vi "Save Control__A2E.vi"(8 "error in (no error)":errorcluster, 10 "Control VI Type":T1, 11 "vi reference in":refnum<vi>) -> (0 "error out":errorcluster, 3 "vi reference out":refnum<vi>)   [LabVIEW 2021, in "Utilities.lvlib"]
uses:
  ControlTypes__A2E.ctl
  Utilities.lvlib
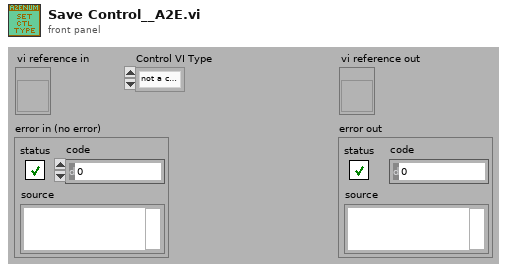
[diagram p1: front panel]
types:
  T1 = typedef "Utilities.lvlib/ControlTypes__A2E.ctl" = enum32{"not a control VI", "control", "typedef", "strict typedef"}
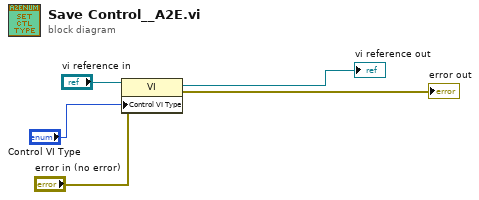
[diagram p0: block diagram]
diagram:
  n1 = property class="VI"(reference="vi reference in", error in="error in (no error)", "Control VI Type"="Control VI Type") -> (reference out=→"vi reference out":refnum<vi>, error out=→"error out":errorcluster)
